vi "Read Digital Port.vi"(8 "error in (no error)":errorcluster, 11 "Digital Input in":refnum<class "DI.lvclass">) -> (0 "error out":errorcluster, 2 "DIs":bool[](array[boolean]), 3 "Digital Input out":refnum<class "DI.lvclass">)   [LabVIEW 2025, in "Interface.lvlib" / "DI.lvclass"]
uses:
  DI.lvclass
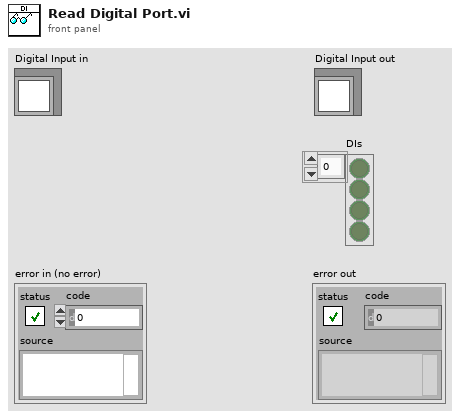
[diagram p1: front panel]
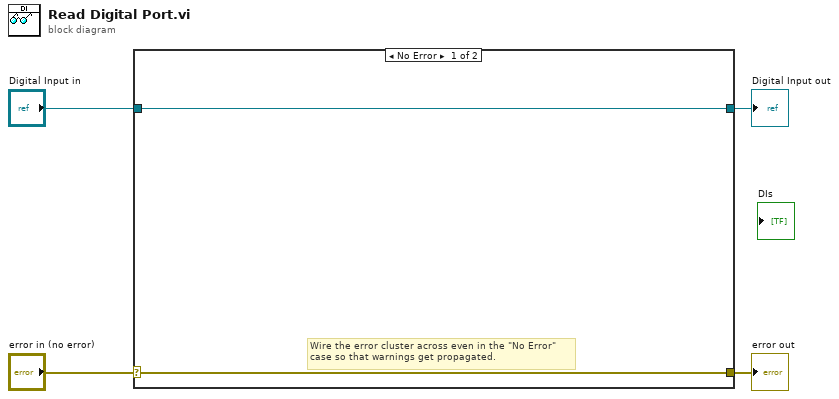
[diagram p0: block diagram]
diagram:
  n1 = case shown="No Error" "error in (no error)" {
    selector: "error in (no error)" -> [w5 w8]
    tunnel: [w5 w8] -> w3
    tunnel: [w6 w7] -> w1
    tunnel: "Digital Input in" -> [w6 w7]
    frame No Error {
      # "Wire the error cluster across even in the \"No Error\"\ncase so that warnings get propagated."
    }
    frame Error {
    }
  }
  "error out" <- w3
  "Digital Input out" <- w1
